vi "Build API Map.vi"(1 "DAQmx IO Folder":string) -> (0 "API map":map{T1, map{T2, string}}(c390))   [LabVIEW 2021, in "Acquisition.lvlib"]
doc: "Build a map of API calls for each supported API."
uses:
  Acquisition.lvlib
  IO API.ctl
  API Call.ctl
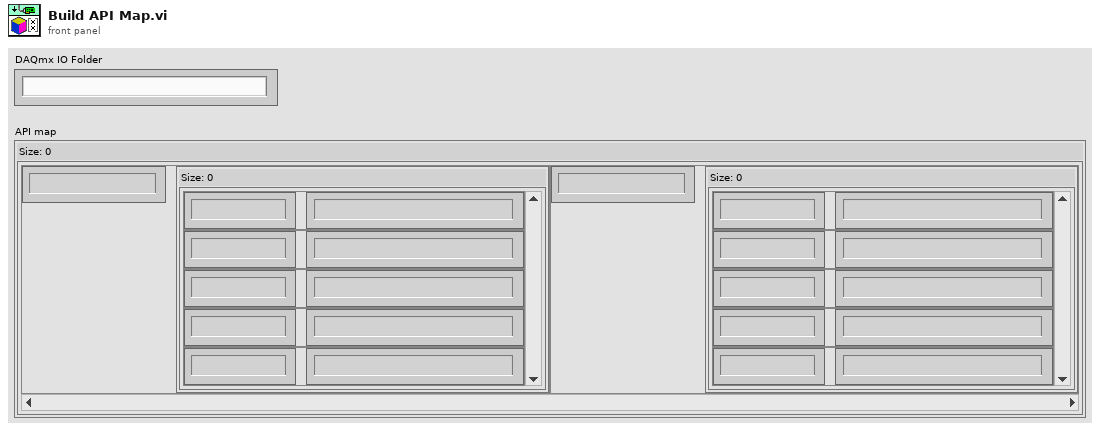
[diagram p1: front panel]
types:
  T1 = typedef "Acquisition.lvlib/IO API.ctl" = enum16{"Simulated", "DAQmx"}
  T2 = typedef "Acquisition.lvlib/API Call.ctl" = enum16{"On Start", "Acquire", "On Stop", "Preview"}
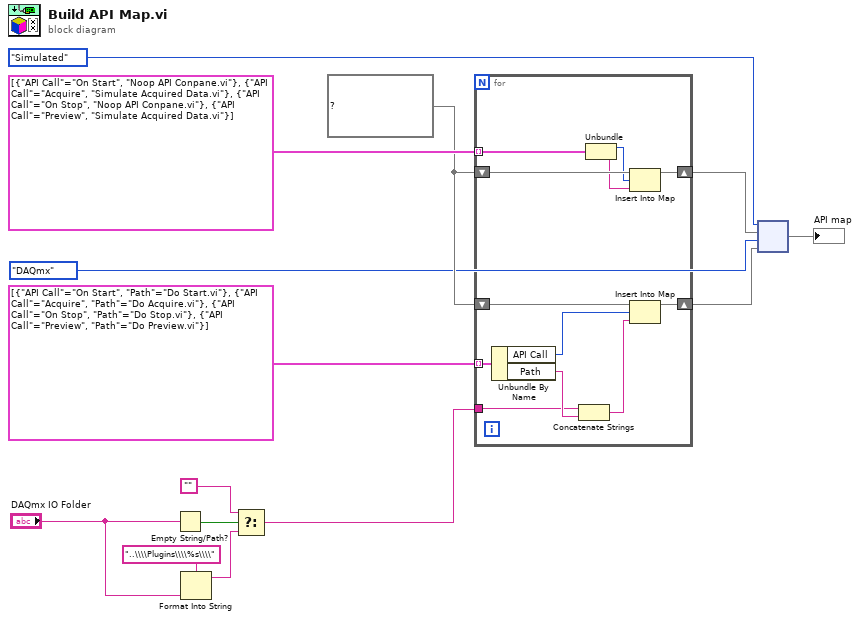
[diagram p0: block diagram]
diagram:
  w12 = map{T2, string} {} ("map")
  n1 = Empty String/Path?(string/path="DAQmx IO Folder") -> (empty?=w6:bool)
  n2 = Format Into String(format string="..\\\\Plugins\\\\%s\\\\", "DAQmx IO Folder") -> (resulting string=w1:string)  [unwired: 2 in, 1 out]
  n3 = Select(t="", s=w6, f=w1) -> (s? t:f=w4:string)
  n4 = for {
    tunnel: cluster{"API Call":T2, string}[] [{"API Call"=enum."On Start", "Noop API Conpane.vi"}, {"API Call"=enum."Acquire", "Simulate Acquired Data.vi"}, {"API Call"=enum."On Stop", "Noop API Conpane.vi"}, {"API Call"=enum."Preview", "Simulate Acquired Data.vi"}] -> [w26] mode=indexing
    shift-right: [w22] -> w10
    shift-left: w12 -> [w25]
    tunnel: cluster{"API Call":T2, "Path":string}[] [{"API Call"=enum."On Start", "Path"="Do Start.vi"}, {"API Call"=enum."Acquire", "Path"="Do Acquire.vi"}, {"API Call"=enum."On Stop", "Path"="Do Stop.vi"}, {"API Call"=enum."Preview", "Path"="Do Preview.vi"}] -> [w19] mode=indexing
    shift-right: [w20] -> w8
    shift-left: w12 -> [w21]
    tunnel: w4 -> [w15]
    n5 = Unbundle By Name(w19) -> ("API Call"=w18:T2, "Path"=w17:string)
    n6 = Concatenate Strings(w15, w17) -> (w16:string)
    n7 = Unbundle(w26) -> ("API Call"=w24:T2, w23:string)
    n8 = Insert Into Map(map in=w25, key=w24, value=w23) -> (map out=w22:map{T2, string})  [unwired: 2 out]
    n9 = Insert Into Map(map in=w21, key=w18, value=w16) -> (map out=w20:map{T2, string})  [unwired: 2 out]
  }
  n10 = node(IO_API."Simulated" ("API"), w10, IO_API."DAQmx" ("API"), w8) -> (→"API map":map{T1, map{T2, string}})
